vi "Move Axis.vi"(8 "error in (no error)":errorcluster, 10 "Position":dbl, 11 "Axis":i32) -> (0 "error out":errorcluster)   [LabVIEW 2020, in "Manipulator CLI Driver.lvlib"]
uses:
  Manipulator CLI Driver.lvlib
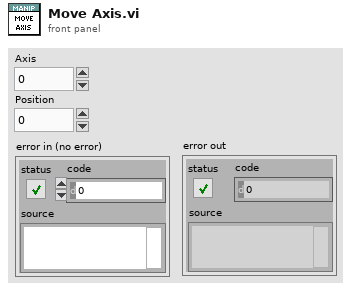
[diagram p1: front panel]
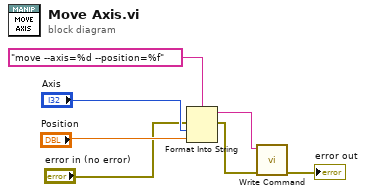
[diagram p0: block diagram]
diagram:
  n1 = Format Into String(format string="move --axis=%d --position=%f", error in="error in (no error)", "Axis", "Position") -> (resulting string=w3:string, error out=w1:errorcluster)  [unwired: 1 in]
  n2 = call "Write Command.vi"("error in (no error)"=w1, "command"=w3) -> ("error out"=→"error out":errorcluster)  [unwired: 7 in, 2 out]
